vi "DACTest.vi"() -> ()   [LabVIEW 2011]
uses:
  <vilib>/LabVIEW Interface for Arduino/Type Defs/SPI Bit Order.ctl
  <vilib>/LabVIEW Interface for Arduino/Type Defs/SPI Clock Divider.ctl
  <vilib>/LabVIEW Interface for Arduino/Type Defs/SPI Data Mode.ctl
  <vilib>/LabVIEW Interface for Arduino/Type Defs/Pin Mode.ctl
  <vilib>/LabVIEW Interface for Arduino/LabVIEW Interface for Arduino.lvlib
panel:
  out "Impedance":dbl(graph)
  in  "Remove Button":bool
  out "Signals":T1(graph)
  in  "Brightness":dbl(slide) scale=0.0..100.0
  in  "Stop Button":bool
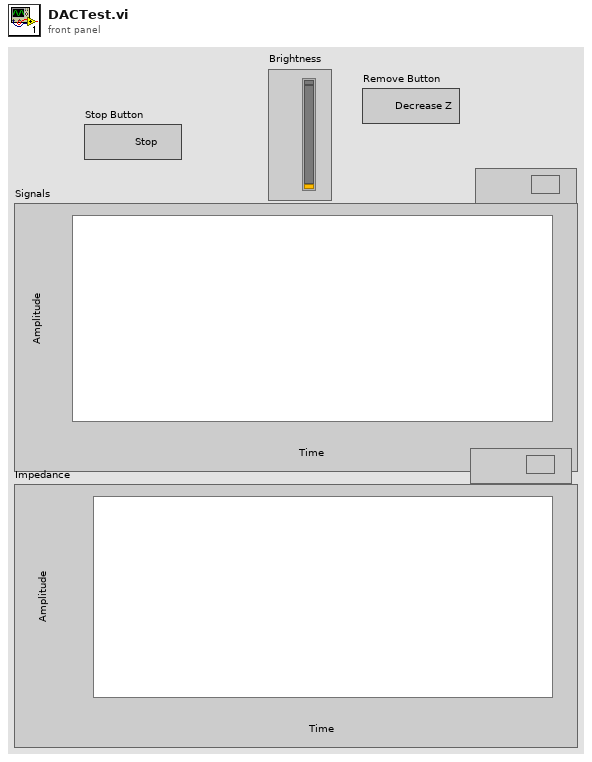
[diagram p1: front panel]
types:
  T1 = cluster{"Numeric":dbl, "Numeric":dbl, "Numeric":dbl, "Numeric":dbl, "Numeric":dbl}
  T2 = typedef "LabVIEW Interface for Arduino.lvlib/Pin Mode.ctl" = enum8{"Input", "Output"}
  T3 = typedef "LabVIEW Interface for Arduino.lvlib/SPI Data Mode.ctl" = enum8{"Mode 0", "Mode 1", "Mode 2", "Mode 3"}
  T4 = typedef "LabVIEW Interface for Arduino.lvlib/SPI Clock Divider.ctl" = enum8{"2", "4", "8", "16", "32", "64", "128"}
  T5 = typedef "LabVIEW Interface for Arduino.lvlib/SPI Bit Order.ctl" = enum8{"LSB First", "MSB First"}
  T6 = typedef "LabVIEW Interface for Arduino.lvlib/Arduino Resource.ctl" = cluster{"VISA resource":refnum<visa-resource-name>, "Board Type":T7, "Connection Type":enum8{"USB / Serial"}, "Bytes Per Packet (15)":u8}
  T7 = typedef "LabVIEW Interface for Arduino.lvlib/Board Type.ctl" = enum16{"Uno", "Dimuelanove w/Atmega 328", "Mega 2560"}
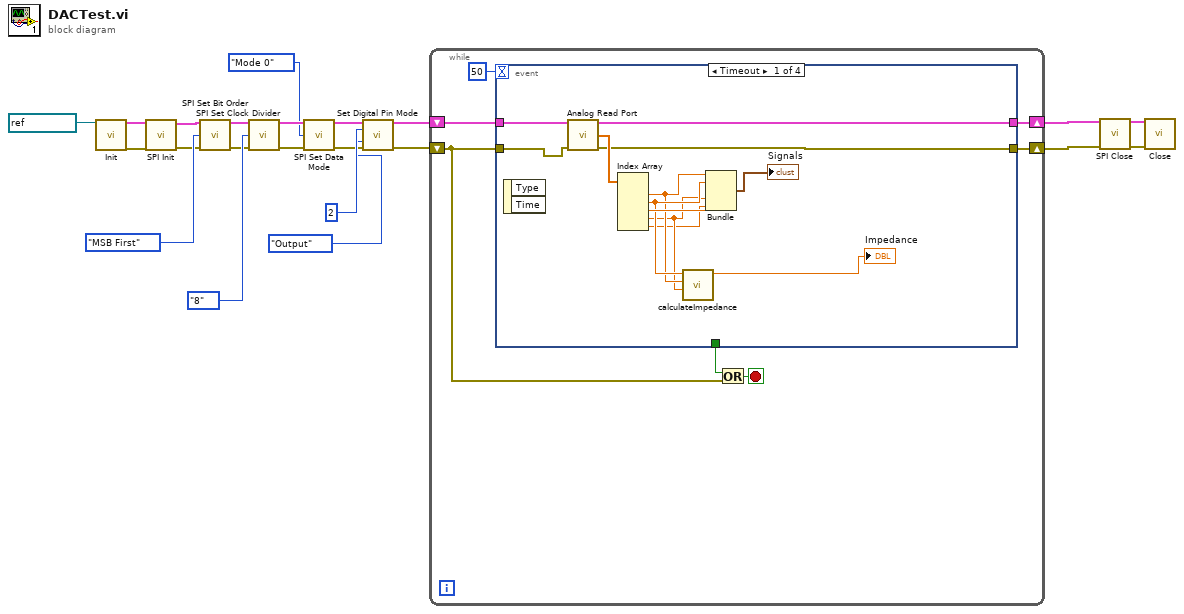
[diagram p0: block diagram]
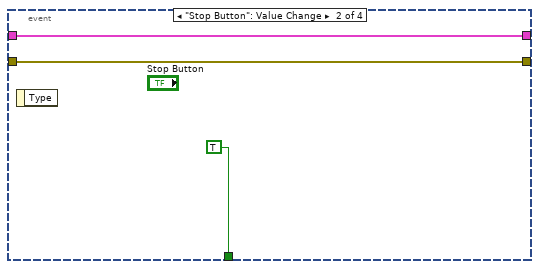
[diagram p2: hidden frame]
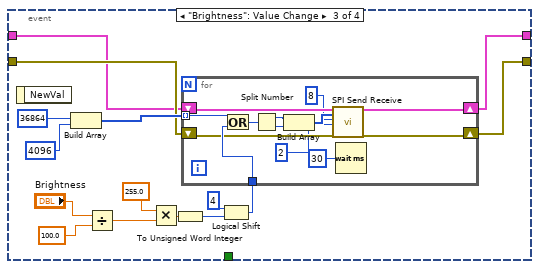
[diagram p3: hidden frame]
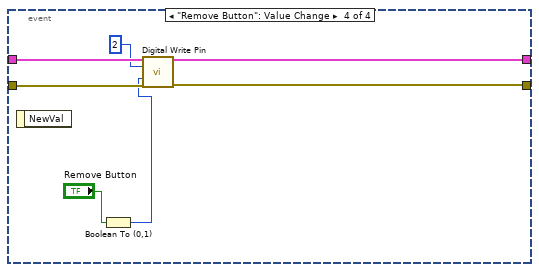
[diagram p4: hidden frame]
diagram:
  n1 = call <vilib>:"Init.vi"("VISA resource"=refnum<visa-resource-name> "COM14") -> ("Arduino Resource"=w22:T6, "error out"=w21:errorcluster)  [unwired: 17 in]
  n2 = call <vilib>:"SPI Init.vi"("error in"=w21, "Arduino Resource"=w22) -> ("error out"=w18:errorcluster, "Arduino Resource"=w19:T6)  [unwired: 8 in]
  n3 = call <vilib>:"SPI Set Bit Order.vi"("Arduino Resource"=w19, "SPI Bit Order"=SPI_Bit_Order."MSB First", "error in"=w18) -> ("Arduino Resource"=w16:T6, "error out"=w15:errorcluster)  [unwired: 11 in]
  n4 = call <vilib>:"SPI Set Clock Divider.vi"("Arduino Resource"=w16, "SPI Clock Divider"=SPI_Clock_Divider."8", "error in"=w15) -> ("Arduino Resource"=w14:T6, "error out"=w13:errorcluster)  [unwired: 11 in]
  n5 = call <vilib>:"SPI Set Data Mode.vi"("Arduino Resource"=w14, "SPI Data Mode"=SPI_Data_Mode."Mode 0", "error in"=w13) -> ("Arduino Resource"=w5:T6, "error out"=w4:errorcluster)  [unwired: 11 in]
  n6 = call <vilib>:"Set Digital Pin Mode.vi"("Arduino Resource"=w5, "Digital I/O Pin"=u8 2, "Pin Mode (Input)"=Pin_Mode."Output", "error in"=w4) -> ("Arduino Resource"=w2:T6, "error out"=w3:errorcluster)  [unwired: 10 in]
  n7 = while {
    shift-right: [w29] -> w11
    shift-left: w2 -> [w23]
    shift-right: [w25] -> w10
    shift-left: w3 -> [w26]
    stop <- w27 stop-if-true
    n8 = event shown="[0] Timeout" {
      selector: _ -> [_ _ _ _]
      dyn-events: _ -> [_ _ _ _]
      timeout: 50 -> [_ _ _ _]
      tunnel: [_ TRUE _ _] -> w28
      tunnel: w23 -> [w38 w43 w47 w79]
      tunnel: [w35 w43 w46 w74] -> w29
      tunnel: w26 -> [w37 w42 w48 w78]
      tunnel: [w36 w42 w45 w73] -> w25
      event Timeout {
        n9 = event-data() -> ()  [unwired: 1 in, 2 out]
        n10 = call <vilib>:"Analog Read Port.vi"("Arduino Resource"=w38, "error in"=w37) -> ("Arduino Resource"=w35:T6, "Analog Port"=w41:dbl[], "error out"=w36:errorcluster)  [unwired: 11 in]
        n11 = Index Array(array=w41) -> (element #1=w32:dbl, element #2=w34:dbl, element #3=w40:dbl, element #4=w31:dbl, element #5=w30:dbl)  [unwired: 5 in]
        n12 = call "calculateImpedance.vi"("Vmeas"=w31, "Vb"=w32, "V"=w34) -> ("Z"=→"Impedance":dbl)  [unwired: 8 in]
        n13 = Bundle("Numeric"=w32, "Numeric"=w34, "Numeric"=w40, "Numeric"=w31, "Numeric"=w30) -> (→"Signals":T1)  [unwired: 1 in]
      }
      event "Stop Button": Value Change {
        n14 = event-data() -> ()  [unwired: 1 in, 1 out]
      }
      event "Brightness": Value Change {
        n15 = event-data() -> ()  [unwired: 1 in, 1 out]
        n16 = Build Array(u16 36864, u16 4096) -> (w52:u16[])
        n17 = Divide(x="Brightness", y=100.0) -> (x/y=w57:dbl)
        n18 = Multiply(x=255.0, y=w57) -> (x*y=w55:dbl)
        n19 = To Unsigned Word Integer(number=w55) -> (unsigned 16bit integer=w51:u16)
        n20 = Logical Shift(y=i8 4, x=w51) -> (x << y=w49:u16)
        n21 = for {
          tunnel: w52 -> [w72] mode=indexing
          tunnel: w49 -> [w71]
          shift-right: [w61] -> w45
          shift-left: w48 -> [w65]
          shift-right: [w60] -> w46
          shift-left: w47 -> [w66]
          n22 = Or(x=w72, y=w71) -> (x .or. y?=w70:u16)
          n23 = Split Number(x=w70) -> (hi(x)=w69:u8, lo(x)=w68:u8)
          n24 = Build Array(w69, w68) -> (w67:u8[])
          n25 = call <vilib>:"SPI Send Receive.vi"("Arduino Resource"=w66, "SPI Data"=w67, "Chip Select DIO Pin"=u8 8, "Word Size (Bytes)"=u8 2, "error in"=w65) -> ("Arduino Resource"=w60:T6, "error out"=w61:errorcluster)  [unwired: 12 in, 1 out]
          n26 = Wait (ms)(milliseconds to wait=u32 30) -> ()  [unwired: 1 out]
        }
      }
      event "Remove Button": Value Change {
        n27 = event-data() -> ()  [unwired: 1 in, 1 out]
        n28 = Boolean To (0,1)(Boolean="Remove Button") -> (0, 1=w76:i16)
        n29 = call <vilib>:"Digital Write Pin.vi"("Arduino Resource"=w79, "Digital I/O Pin (0)"=u8 2, "Value (0)"=w76, "error in"=w78) -> ("Arduino Resource"=w74:T6, "error out"=w73:errorcluster)  [unwired: 10 in]
      }
    }
    n30 = Or(x=w28, y=w26) -> (x .or. y?=w27:bool)
  }
  n31 = call <vilib>:"SPI Close.vi"("Arduino Resource"=w11, "error in"=w10) -> ("Arduino Resource"=w8:T6, "error out"=w9:errorcluster)  [unwired: 12 in]
  n32 = call <vilib>:"Close.vi"("Arduino Resource"=w8, "error in"=w9) -> ()  [unwired: 13 in, 1 out]
